vi "testPython.vi"(8 "error in (no error)":errorcluster, 11 "reference in":refnum<class "GUI Controller.lvclass">) -> (0 "error out":errorcluster, 3 "reference out":refnum<class "GUI Controller.lvclass">)   [LabVIEW 2015, in "GUI Controller.lvclass"]
uses:
  GUI Controller.lvclass
  Project Panels_class/Project Panels.lvclass
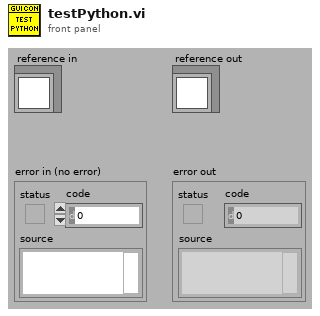
[diagram p1: front panel]
types:
  T1 = typedef "GUI Controller.lvclass/ObjectAttributesRef.ctl" = refnum<data-value>
  T2 = typedef "GUI Controller.lvclass/ObjectAttributes.ctl" = cluster{"MyAttribute":dbl, "state":T3, "project_panels_ref":refnum<class "Project Panels.lvclass">, "items_controller_ref":refnum<class "Items Controller.lvclass">, "notification_controller_ref":refnum<class "Notification Controller.lvclass">, "partstracking_controller_ref":refnum<class "PartsTracking Controller.lvclass">, "file_controller_ref":refnum<class "File Controller.lvclass">, "low_resolution?":bool, "run_python?":bool}
  T3 = typedef "GUI Controller.lvclass/state.ctl" = enum16{"initiate", "checkNotificationItems", "checkNotificationTracking", "operate", "updateFromFile", "stop"}
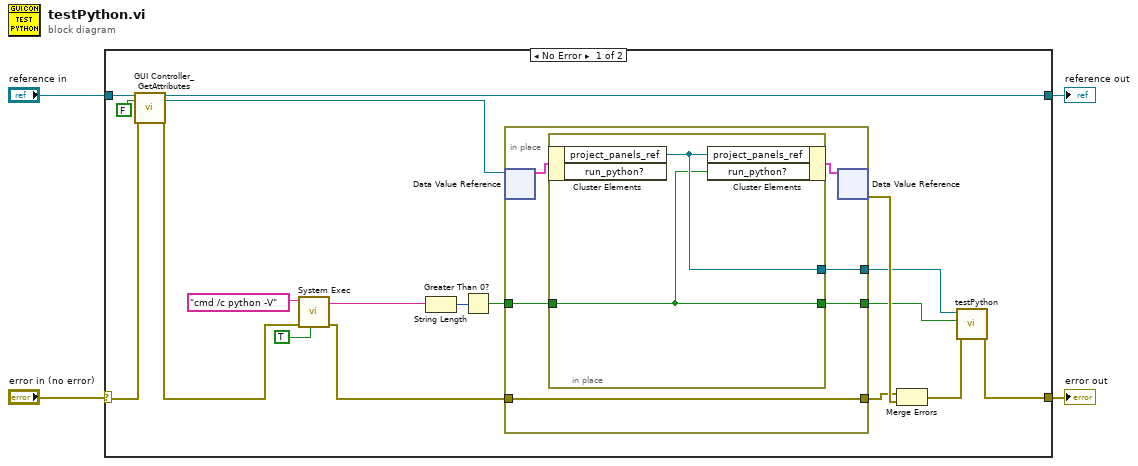
[diagram p0: block diagram]
diagram:
  n1 = case shown="No Error" "error in (no error)" {
    selector: "error in (no error)" -> [w18 w32]
    tunnel: [w14 w32] -> w3
    tunnel: [w17 w31] -> w1
    tunnel: "reference in" -> [w20 w31]
    frame No Error {
      n2 = call "GUI Controller_GetAttributes.vi"("reference in"=w20, "return data? (T)"=FALSE, "error in (no error)"=w18) -> ("reference out"=w17:refnum<class "GUI Controller.lvclass">, "attributes ref"=w16:T1, "error out"=w7:errorcluster)  [unwired: 13 in, 1 out]
      n3 = call <vilib>:"System Exec.vi"("run minimized? (F)"=TRUE, "error in (no error)"=w7, "command line"="cmd /c python -V") -> ("error out"=w6:errorcluster, "standard output"=w9:string)  [unwired: 3 in, 4 out]
      n4 = String Length(string=w9) -> (length=w8:i32)
      n5 = Greater Than 0?(x=w8) -> (x > 0?=w5:bool)
      n6 = in-place {
        in-place-border: w6 -> [w26]
        in-place-border: [w26] -> w21
        in-place-border: w5 -> [w25]
        in-place-border: [w24] -> w13
        in-place-border: [w23] -> w12
        n7 = in-place-dvr #1(w16) -> (w27:T2)  [unwired: 1 out]
        n8 = in-place {
          in-place-border: w25 -> [w29]
          in-place-border: [w30] -> w24
          in-place-border: [w29] -> w23
          n9 = in-place-cluster #2(w27) -> ("project_panels_ref"=w30:refnum<class "Project Panels.lvclass">)  [unwired: 1 out]
          n10 = in-place-cluster #2("project_panels_ref"=w30, "run_python?"=w29) -> (w28:T2)
        }
        n11 = in-place-dvr #1(w28) -> (w22:errorcluster)  [unwired: 1 out]
      }
      n12 = Merge Errors(w21, w22) -> (w15:errorcluster)
      n13 = call "testPython.vi"("error in (no error)"=w15, "run_python?"=w12, "reference in"=w13) -> ("error out"=w14:errorcluster)  [unwired: 7 in, 1 out]
    }
    frame Error {
    }
  }
  "error out" <- w3
  "reference out" <- w1
